vi "Field_Init_AMI.vi"   [LabVIEW 2016]
uses:
  Global/Global Variables/global.vi
  Global/Global Variables/Data_Display_global.vi
types:
  T1 = enum16{"", "RAMPING", "HOLDING", "PAUSED", "MANUAL UP", "MANUAL DOWN", "ZEROING CURRENT", "QUENCH DETECTED", "HEATING SWITCH", "AT ZER0", "COOLING SWITCH"}
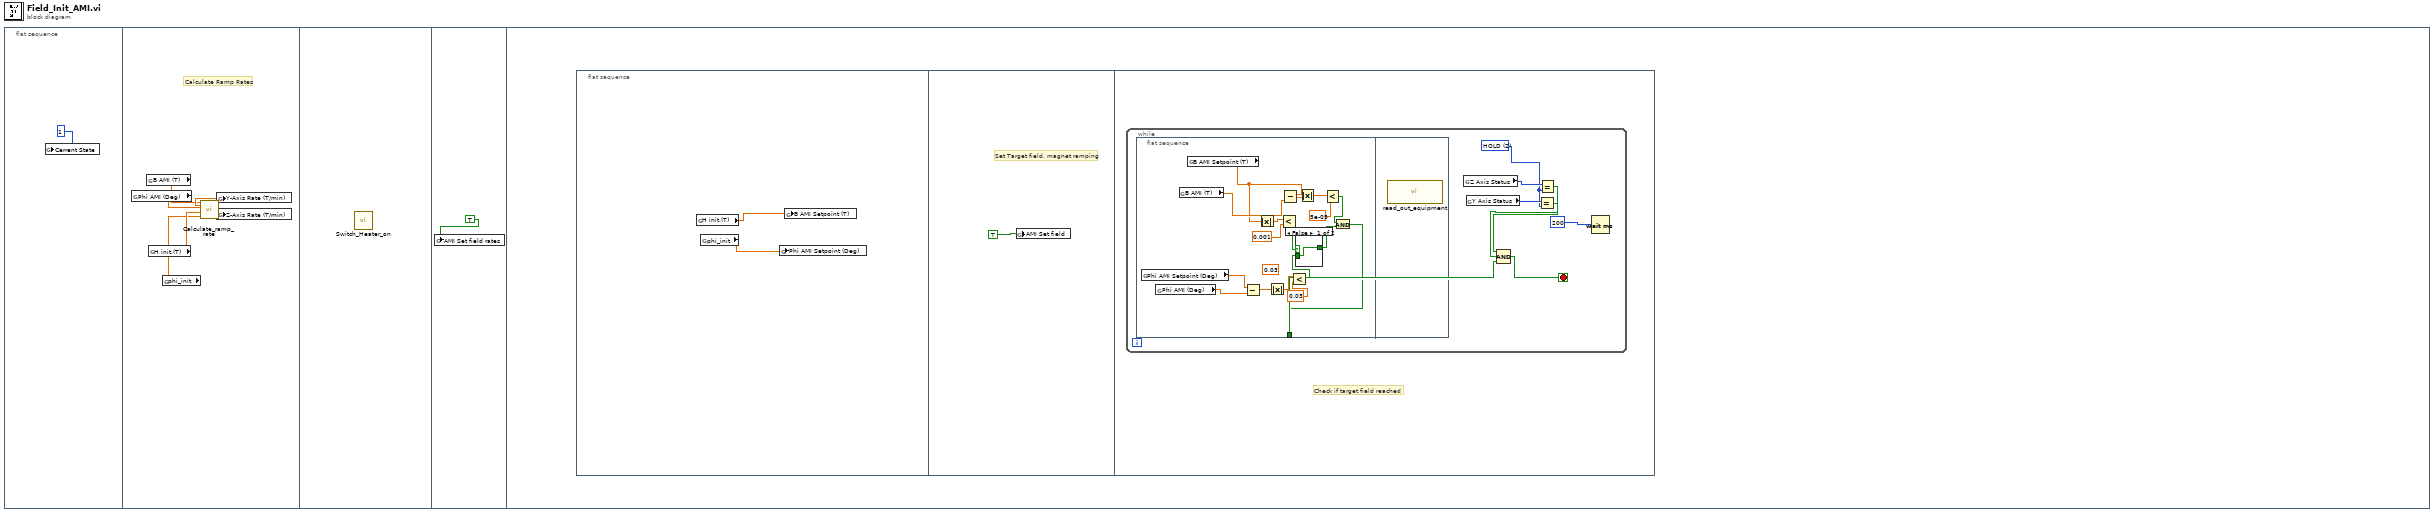
[diagram p0: block diagram]
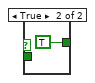
[diagram p2: hidden frame]
diagram:
  n1 = flat-sequence {
    frame #0 {
      n2 = global write "global.vi" "Cerrent State"(1) -> ()
    }
    frame #1 {
      # "Calculate Ramp Rates"
      n3 = global read "Data_Display_global.vi" "Phi AMI (Deg)"() -> (w5:dbl)
      n4 = global read "Data_Display_global.vi" "B AMI (T)"() -> (w4:dbl)
      n5 = global read "global.vi" "H init.(T)"() -> (w3:dbl)
      n6 = global read "global.vi" "phi_init"() -> (w2:dbl)
      n7 = call "Calculate_ramp_rate.vi"("Phi (Deg)"=w2, "H_final (T)"=w3, "Phi_init (Deg)"=w5, "H_init (T)"=w4) -> ("Z-Ramp"=w6:dbl, "Y-Ramp"=w7:dbl)  [unwired: 2 in]
      n8 = global write "Data_Display_global.vi" "Y-Axis Rate (T/min)"(w7) -> ()
      n9 = global write "Data_Display_global.vi" "Z-Axis Rate (T/min)"(w6) -> ()
    }
    frame #2 {
      n10 = call "Switch_Heater_on.vi"() -> ()  [unwired: 12 in]
    }
    frame #3 {
      n11 = global write "Data_Display_global.vi" "AMI Set field rates"(TRUE) -> ()
    }
    frame #4 {
      n12 = flat-sequence {
        frame #0 {
          n13 = global read "global.vi" "H init.(T)"() -> (w10:dbl)
          n14 = global read "global.vi" "phi_init"() -> (w9:dbl)
          n15 = global write "Data_Display_global.vi" "Phi AMI Setpoint (Deg)"(w9) -> ()
          n16 = global write "Data_Display_global.vi" "B AMI Setpoint (T)"(w10) -> ()
        }
        frame #1 {
          # "Set Target field, magnet ramping"
          n17 = global write "Data_Display_global.vi" "AMI Set field"(TRUE) -> ()
        }
        frame #2 {
          # "Check if target field reached"
          n18 = while {
            stop <- w13 stop-if-true
            w12 = u16 2 items=["RAMP"=1, "HOLD"=2, "Paused"=3, "Manual Up"=4, "Manual Down"=5, "Zeroing Current"=6, "Quench Detected"=7, "At Zero"=8, "Heating Switch"=9, "Cooling Switch "=10] ("Ramping Mode")
            n19 = flat-sequence {
              tunnel: [w26] -> w14
              frame #0 {
                (unwired) 0.03 ("y")
                n20 = global read "Data_Display_global.vi" "Phi AMI Setpoint (Deg)"() -> (w29:dbl)
                n21 = global read "Data_Display_global.vi" "Phi AMI (Deg)"() -> (w28:dbl)
                n22 = global read "Data_Display_global.vi" "B AMI (T)"() -> (w33:dbl)
                n23 = global read "Data_Display_global.vi" "B AMI Setpoint (T)"() -> (w20:dbl)
                n24 = Subtract(x=w29, y=w28) -> (x-y=w30:dbl)
                n25 = Absolute Value(x=w20) -> (abs(x)=w25:dbl)
                n26 = Absolute Value(x=w30) -> (abs(x)=w31:dbl)
                n27 = Less?(x=w25, y=0.001) -> (x < y?=w23:bool)
                n28 = Subtract(x=w20, y=w33) -> (x-y=w35:dbl)
                n29 = Less?(x=w31, y=0.03) -> (x < y?=w21:bool)
                n30 = case shown="False" w23 {
                  tunnel: [w37 TRUE] -> w22
                  tunnel: w21 -> [w37 _]
                  frame False {
                  }
                  frame True {
                  }
                }
                n31 = Absolute Value(x=w35) -> (abs(x)=w34:dbl)
                n32 = Less?(x=w34, y=5e-05) -> (x < y?=w27:bool)
                n33 = And(x=w27, y=w22) -> (x .and. y?=w26:bool)
              }
              frame #1 {
                n34 = call "read_out_equipment.vi"() -> ()  [unwired: 1 in]
              }
            }
            n35 = global read "Data_Display_global.vi" "Z Axis Status"() -> (w18:T1)
            n36 = global read "Data_Display_global.vi" "Y Axis Status"() -> (w17:T1)
            n37 = Equal?(x=w17, y=w12) -> (x = y?=w15:bool)
            n38 = Equal?(x=w18, y=w12) -> (x = y?=w16:bool)
            n39 = Compound Arithmetic op=AND(w16, w15, w14) -> (w13:bool)
            n40 = Wait (ms)(milliseconds to wait=200) -> ()  [unwired: 1 out]
          }
        }
      }
    }
  }
